vi "Image Display Get-Set ROI.vi"(6 "Get(F)/Set":bool, 8 "Error In":errorcluster, 10 "ROI Descriptor in":T2 {"Contours"."Type" items=["No Selection", "Point", "Line", "Rectangle", "Oval", "Polygon", "Freehand Region", "Annulus", "Unused2", "Unused3", "Broken Line", "Freehand Line", "Rotated Rectangle"]}, 11 "Image Display Refnum":T1 caption="Source Image Display Refnum") -> (0 "Error Out":errorcluster, 1 "Label.Text":string, 2 "ROI Descriptor out":T2 {"Contours"."Type" items=["No Selection", "Point", "Line", "Rectangle", "Oval", "Polygon", "Freehand Region", "Annulus", "Unused2", "Unused3", "Broken Line", "Freehand Line", "Rotated Rectangle"]}, 3 "Image Display Refnum (dup)":T1 caption="Source Image Display Refnum", 4 "CPU (s)":dbl)   [LabVIEW 2021, in "Image.lvlib"]
uses:
  Image.lvlib
  Image Control Refnum.ctl
  Time/Time.lvlib
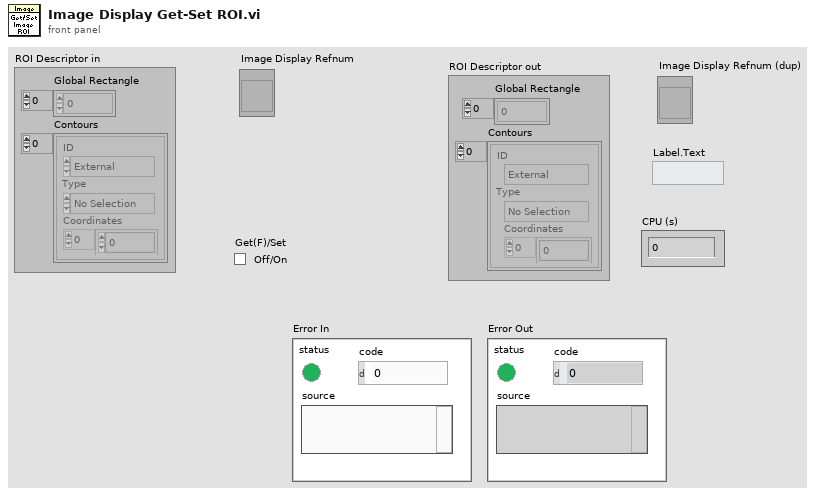
[diagram p1: front panel]
types:
  T1 = typedef "Image.lvlib/Image Control Refnum.ctl" = refnum<vi>
  T2 = typedef "ROI Descriptor" = cluster{"Global Rectangle":i32[], "Contours":cluster{"ID":enum32{"External", "Internal"}, "Type":u32, "Coordinates":i32[]}[]}
  T3 = cluster{"Global Rectangle":i32[], "Contours":cluster{"Contour Type":u32, "ROI Type":u32, "Points":i32[]}[]}
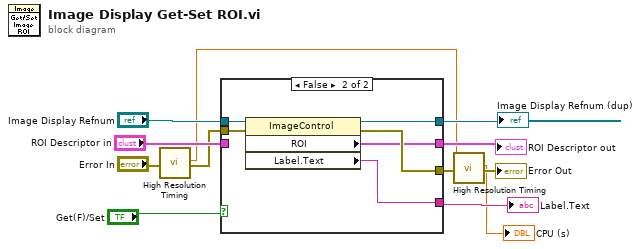
[diagram p0: block diagram]
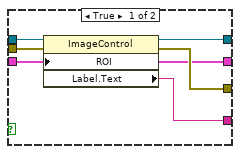
[diagram p2: hidden frame]
diagram:
  n1 = call "High Resolution Timing.vi"("Error In"="Error In") -> ("elapsed (relative) seconds"=w2:dbl, "Error Out"=w4:errorcluster)  [unwired: 16 in, 1 out]
  n2 = case shown="False" "Get(F)/Set" {
    tunnel: "Image Display Refnum" -> [w18 w24]
    tunnel: [w17 w23] -> w11
    tunnel: w4 -> [w16 w22]
    tunnel: "ROI Descriptor in" -> [w15 _]
    tunnel: [w15 w21] -> w7
    tunnel: [w14 w20] -> w6
    tunnel: [w13 w19] -> w5
    frame True {
      n3 = property class="ImageControl"(reference=w18, error in=w16, "ROI"=w15) -> (reference out=w14:T1, error out=w17:errorcluster, "Label.Text"=w13:string)
    }
    frame False {
      n4 = property class="ImageControl"(reference=w24, error in=w22) -> (reference out=w20:T1, error out=w23:errorcluster, "ROI"=w21:T3, "Label.Text"=w19:string)
    }
  }
  "ROI Descriptor out" <- w7
  "Image Display Refnum (dup)" <- w6
  "Label.Text" <- w5
  n5 = call "High Resolution Timing.vi"("relative seconds (NaN)"=w2, "Error In"=w11) -> ("elapsed (relative) seconds"=→"CPU (s)":dbl, "Error Out"=→"Error Out":errorcluster)  [unwired: 15 in, 1 out]
